vi "VISA  Send Receive.vi"(1 "RDY max wait, ms (-1 = forever)":i32=500, 4 "RDY when up":bool=TRUE, 5 "Data ready bit (-1 - ignore)":i32=-1, 6 "Read terminator":i16, 7 "Read Delay, ms":u32, 8 "error in (no error)":errorcluster, 9 "Receive count":i32=256, 10 "data string in":string, 11 "VISA Resource Name":refnum<visa-resource-name>) -> (0 "error out":errorcluster, 2 "data string out":string, 3 "VISA Resource Name Out":refnum<visa-resource-name>)   [LabVIEW 2019]
panel:
  out "data string in":string
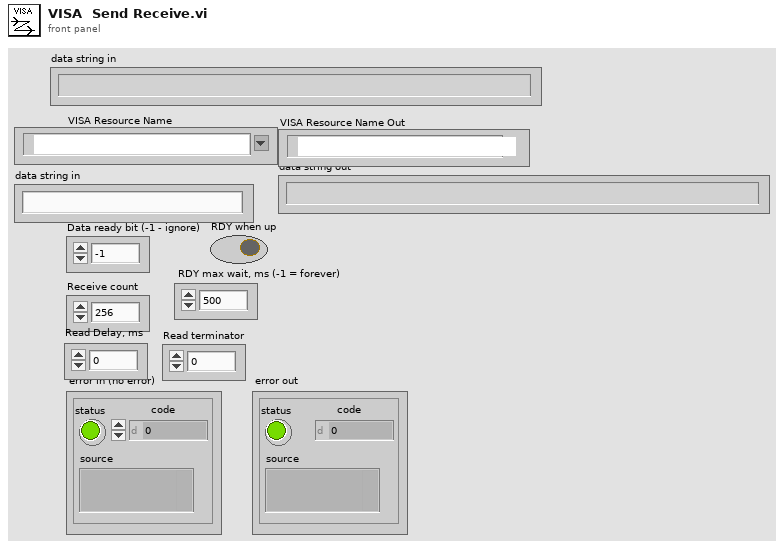
[diagram p1: front panel]
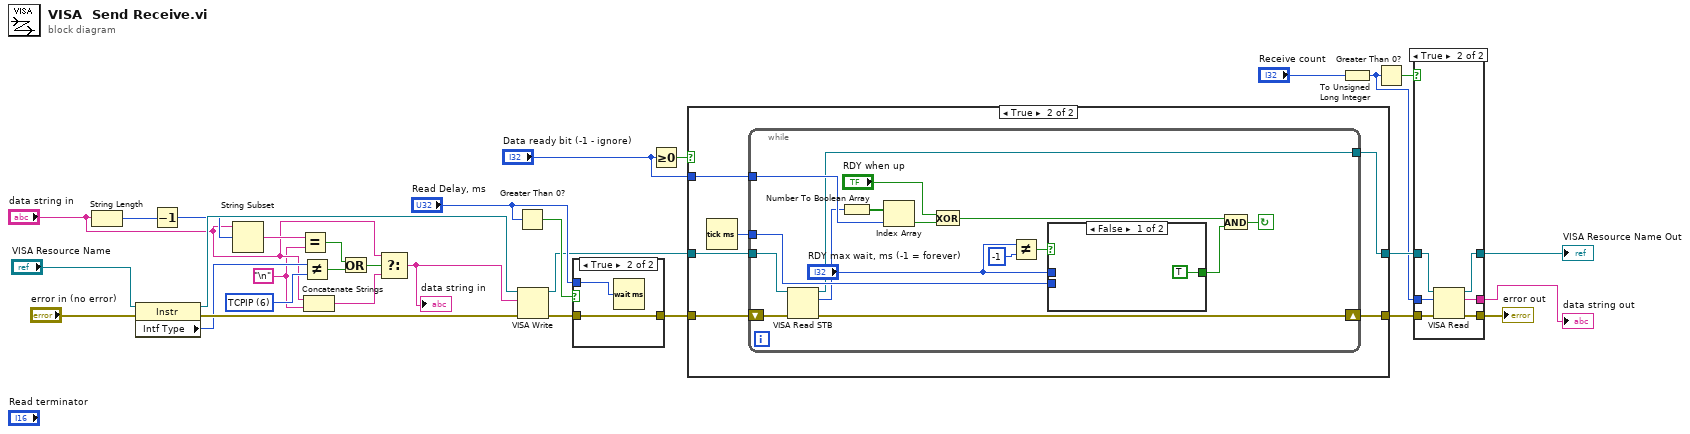
[diagram p0: block diagram]
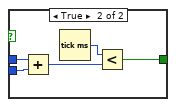
[diagram p4: hidden frame]
diagram:
  w8 = "\n"
  w13 = u16 6 items=["GPIB"=1, "VXI"=2, "GPIB-VXI"=3, "Serial"=4, "PXI"=5, "TCPIP"=6, "USB"=7, "FireWire"=9] ("Interface Information:Interface Type")
  n1 = String Length(string="data string in") -> (length=w12:i32)
  n2 = property class="Instr"(reference="VISA Resource Name", error in="error in (no error)") -> (reference out=w15:refnum<visa-resource-name>, error out=w17:errorcluster, "Intf Type"=w14:u16)
  n3 = Decrement(x=w12) -> (x-1=w11:i32)
  n4 = String Subset(string="data string in", offset (0)=w11) -> (substring=w10:string)  [unwired: 1 in]
  n5 = Equal?(x=w10, y=w8) -> (x = y?=w4:bool)
  n6 = Not Equal?(x=w14, y=w13) -> (x != y?=w5:bool)
  n7 = Concatenate Strings("data string in", w8) -> (w7:string)
  n8 = Or(x=w4, y=w5) -> (x .or. y?=w6:bool)
  n9 = Select(t="data string in", s=w6, f=w7) -> (s? t:f=w1:string)
  "data string in" <- w1
  n10 = Greater Than 0?(x="Read Delay, ms") -> (x > 0?=w29:bool)
  n11 = VISA Write(VISA resource name=w15, write buffer=w1, error in (no error)=w17) -> (VISA resource name out=w22:refnum<visa-resource-name>, error out=w28:errorcluster)  [unwired: 1 out]
  n12 = case shown="True" w29 {
    tunnel: w28 -> [w32 w33]
    tunnel: [w32 w33] -> w25
    tunnel: "Read Delay, ms" -> [_ w34]
    frame False {
    }
    frame True {
      n13 = Wait (ms)(milliseconds to wait=w34) -> ()  [unwired: 1 out]
    }
  }
  n14 = Greater Or Equal To 0?(x="Data ready bit (-1 - ignore)") -> (x >= 0?=w26:bool)
  n15 = case shown="True" w26 {
    tunnel: w25 -> [w36 w41]
    tunnel: "Data ready bit (-1 - ignore)" -> [_ w40]
    tunnel: [w36 w39] -> w23
    tunnel: w22 -> [w35 w38]
    tunnel: [w35 w37] -> w21
    frame False {
    }
    frame True {
      n16 = Tick Count (ms)() -> (millisecond timer value=w42:u32)
      n17 = while {
        shift-right: [w57] -> w39
        shift-left: w41 -> [w58]
        tunnel: w42 -> [w54]
        tunnel: w40 -> [w52]
        tunnel: w38 -> [w48]
        tunnel: [w46] -> w37
        stop <- w56 continue-if-true
        n18 = VISA Read STB(8:w58, 11:w48) -> (0:w57:errorcluster, 2:w47:u16, 3:w46:refnum<visa-resource-name>)
        n19 = Number To Boolean Array(number=w47) -> (Boolean array=w53:bool[])
        n20 = Index Array(array=w53, index=w52) -> (element=w51:bool)
        n21 = Exclusive Or(1:w51, 2:"RDY when up") -> (0:w50:bool)
        n22 = Not Equal?(x="RDY max wait, ms (-1 = forever)", y=-1) -> (x != y?=w45:bool)
        n23 = case shown="False" w45 {
          tunnel: [TRUE w64] -> w55
          tunnel: w54 -> [_ w62]
          tunnel: "RDY max wait, ms (-1 = forever)" -> [_ w60]
          frame False {
          }
          frame True {
            n24 = Add(x=w60, y=w62) -> (x+y=w63:u32)
            n25 = Tick Count (ms)() -> (millisecond timer value=w61:u32)
            n26 = Less?(x=w61, y=w63) -> (x < y?=w64:bool)
          }
        }
        n27 = And(x=w50, y=w55) -> (x .and. y?=w56:bool)
      }
    }
  }
  n28 = To Unsigned Long Integer(number="Receive count") -> (unsigned 32bit integer=w3:u32)
  n29 = Greater Than 0?(x=w3) -> (x > 0?=w2:bool)
  n30 = case shown="True" w2 {
    tunnel: [w66 w72] -> w30
    tunnel: w23 -> [w66 w71]
    tunnel: w21 -> [w65 w70]
    tunnel: w3 -> [_ w69]
    tunnel: [_ w68] -> w19
    tunnel: [w65 w67] -> w18
    frame False {
    }
    frame True {
      n31 = VISA Read(VISA resource name=w70, byte count=w69, error in (no error)=w71) -> (VISA resource name out=w67:refnum<visa-resource-name>, read buffer=w68:string, error out=w72:errorcluster)  [unwired: 1 out]
    }
  }
  "error out" <- w30
  "data string out" <- w19
  "VISA Resource Name Out" <- w18
